vi "Configure TLOG.vi"(0 "VISA resource name":refnum<visa-resource-name>, 1 "Computation Conversion (0 : No Conversion)":i32(ring) items=["No Conversion", "Second", "Minute", "Hour"], 2 "Enable Reset (False)":bool, 5 "Channel (001)":string="001", 7 "Timer Type (0 : Timer)":i32(ring) items=["Timer", "Match Time Timer"], 9 "Timer Number (1)":i32=1 min=1 max=12 step=1, 11 "error in (no error)":errorcluster) -> (4 "VISA resource name out":refnum<visa-resource-name>, 6 "Channel":string, 15 "error out":errorcluster)   [LabVIEW 2020, in "Yokogawa GX Series.lvlib"]
doc: "Sets the TLOG timer.\n\nCommand: STlogMath"
uses:
  <instrlib>/Yokogawa GX Series/Yokogawa GX Series.lvlib
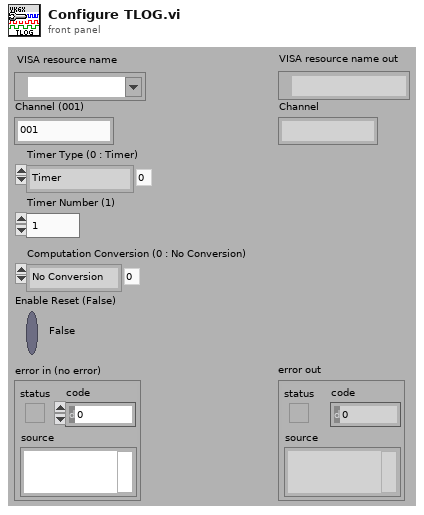
[diagram p1: front panel]
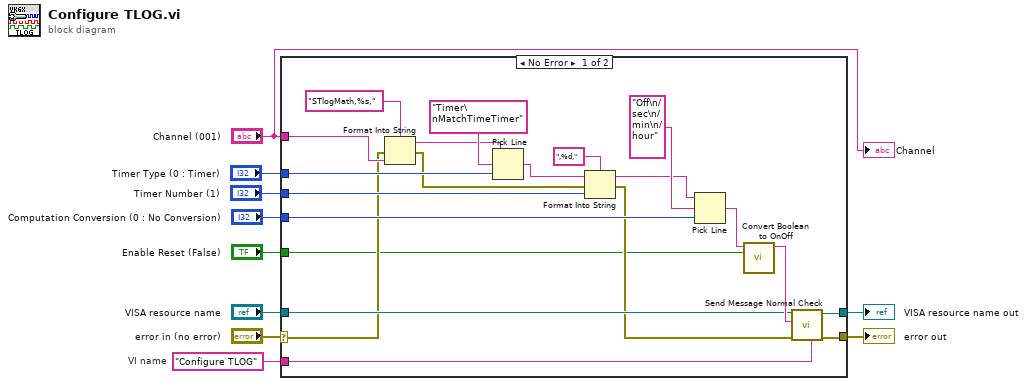
[diagram p0: block diagram]
diagram:
  w9 = "Configure TLOG"  # VI name
  n1 = case shown="No Error" "error in (no error)" {
    selector: "error in (no error)" -> [w12 w32]
    tunnel: "Computation Conversion (0 : No Conversion)" -> [w30 _]
    tunnel: w9 -> [w28 _]
    tunnel: [w27 w33] -> w8
    tunnel: [w26 w32] -> w7
    tunnel: "Timer Type (0 : Timer)" -> [w23 _]
    tunnel: "VISA resource name" -> [w21 w33]
    tunnel: "Timer Number (1)" -> [w17 _]
    tunnel: "Enable Reset (False)" -> [w11 _]
    tunnel: "Channel (001)" -> [w13 _]
    frame No Error {
      n2 = Format Into String(format string="STlogMath,%s,", error in=w12, w13) -> (resulting string=w24:string, error out=w19:errorcluster)  [unwired: 1 in]
      n3 = Pick Line(string ("")=w24, multi-line string="Timer\nMatchTimeTimer", line index=w23) -> (output string=w20:string)
      n4 = Format Into String(format string=",%d,", initial string=w20, error in=w19, w17) -> (resulting string=w16:string, error out=w15:errorcluster)
      n5 = Pick Line(string ("")=w16, multi-line string="Off\n/sec\n/min\n/hour", line index=w30) -> (output string=w14:string)
      n6 = call <instrlib>:"Convert Boolean to OnOff.vi"("On/Off"=w11, "Initial String (\"\")"=w14) -> ("Resulting String"=w22:string)  [unwired: 9 in]
      n7 = call <instrlib>:"Send Message Normal Check.vi"("Source (\"\")"=w28, "error in (no error)"=w15, "Send Message (\"\")"=w22, "VISA resource name"=w21) -> ("error out"=w26:errorcluster, "VISA resource name out"=w27:refnum<visa-resource-name>)  [unwired: 2 in, 4 out]
    }
    frame Error {
    }
  }
  "error out" <- w7
  "VISA resource name out" <- w8
  "Channel" <- "Channel (001)"
